vi "CmdReader with Context.vi"() -> ()   [LabVIEW 2020]
doc: "Copyright © 2008 - 2024 VI Technologies B.V. \nALL RIGHTS RESERVED"
uses:
  <vilib>/dex/Stream Element Allocation Mode.ctl
  SuperNS/SuperNS.lvclass
  MsgData/MsgData.lvclass
panel:
  in  "Connection Config":T2={"BufferSize (100)"=100, "Connection Lost Timeout (2000 ms)"=2000, "Element Allocation Mode"=0, "Low latency mode"=enum."None (High througput mode)", "BG ConnCheck/Read period (200 ms)"=200, "OpenProcessWindow"=TRUE} {"Element Allocation Mode" items=["allocate as needed", "pre-allocate"]}
  in  "Remote EP Config":T3
  in  "Local EP Config":cluster{"Context":string, "Name":string}={"Context"="ReadTestEnv", "Name"="ReaderTest"}
  out "Messages":string
  out "error out":errorcluster
  # "Copyright (c) 2024, VI Technologies B.V.\nAll rights reserved.\n\nRedistribution and use in source and binary forms, with or without modification, are permitted provided that \nthe following conditions are met:\n\n * Redistributions of source code must retain the above copyright notice, this list of conditions and the \nfollowing disclaimer.\n * Redistributions in binary form must reproduce the above copyright notice, this list of conditions and the \nfollowing disclaimer in the documentation and/or other materials provided with the distribution.\n * Neither the name of VI Technologies B.V. nor the names of its contributors may be used to endorse or \npromote products derived from this software without specific prior written permission.\n\nTHIS SOFTWARE IS PROVIDED BY THE COPYRIGHT HOLDERS AND CONTRIBUTORS \"AS IS\" AND ANY EXPRESS OR \nIMPLIED WARRANTIES, INCLUDING, BUT NOT LIMITED TO, THE IMPLIED WARRANTIES OF MERCHANTABILITY \nAND FITNESS FOR A PARTICULAR PURPOSE ARE DISCLAIMED. IN NO EVENT SHALL THE COPYRIGHT OWNER OR \nCONTRIBUTORS BE LIABLE FOR ANY DIRECT, INDIRECT, INCIDENTAL, SPECIAL, EXEMPLARY, OR CONSEQUENTIAL \nDAMAGES (INCLUDING, BUT NOT LIMITED TO, PROCUREMENT OF SUBSTITUTE GOODS OR SERVICES; LOSS OF \nUSE, DATA, OR PROFITS; OR BUSINESS INTERRUPTION) HOWEVER CAUSED AND ON ANY THEORY OF LIABILITY, \nWHETHER IN CONTRACT, STRICT LIABILITY, OR TORT (INCLUDING NEGLIGENCE OR OTHERWISE) ARISING IN ANY \nWAY OUT OF THE USE OF THIS SOFTWARE, EVEN IF ADVISED OF THE POSSIBILITY OF SUCH DAMAGE.\n\nFor more information, please visit https://www.vi-tech.nl or contact us at info@vi-tech.nl"
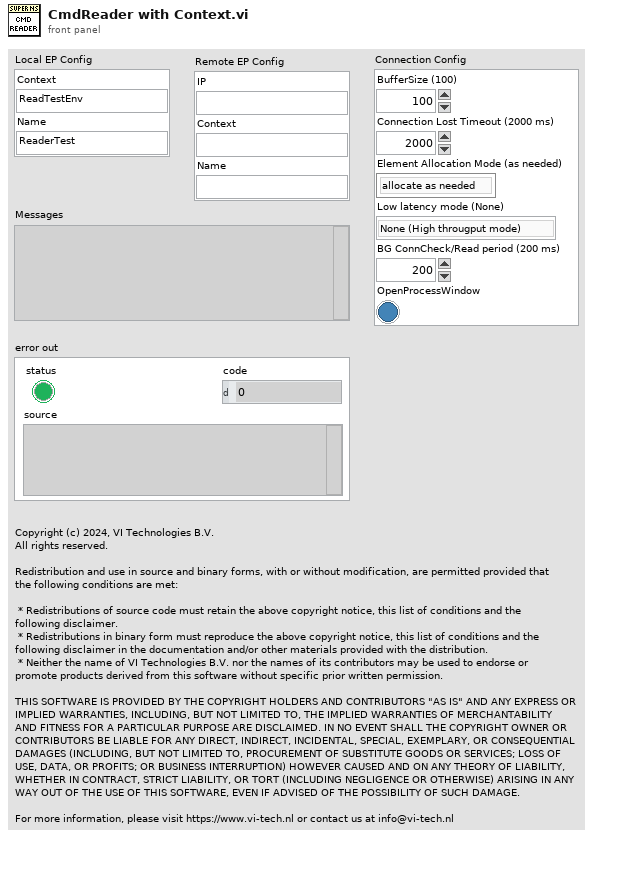
[diagram p1: front panel]
types:
  T1 = typedef "Stream Element Allocation Mode.ctl" = u32
  T2 = cluster{"BufferSize (100)":i32, "Connection Lost Timeout (2000 ms)":i32, "Element Allocation Mode":T1, "Low latency mode":enum16{"None (High througput mode)", "All Elements Read From Stream", "All Elements Available for Reading"}, "BG ConnCheck/Read period (200 ms)":i32, "OpenProcessWindow":bool}
  T3 = cluster{"IP":string, "Context":string, "Name":string}
  T4 = typedef "SuperNS.lvclass/StreamDataType.ctl" = refnum<class>
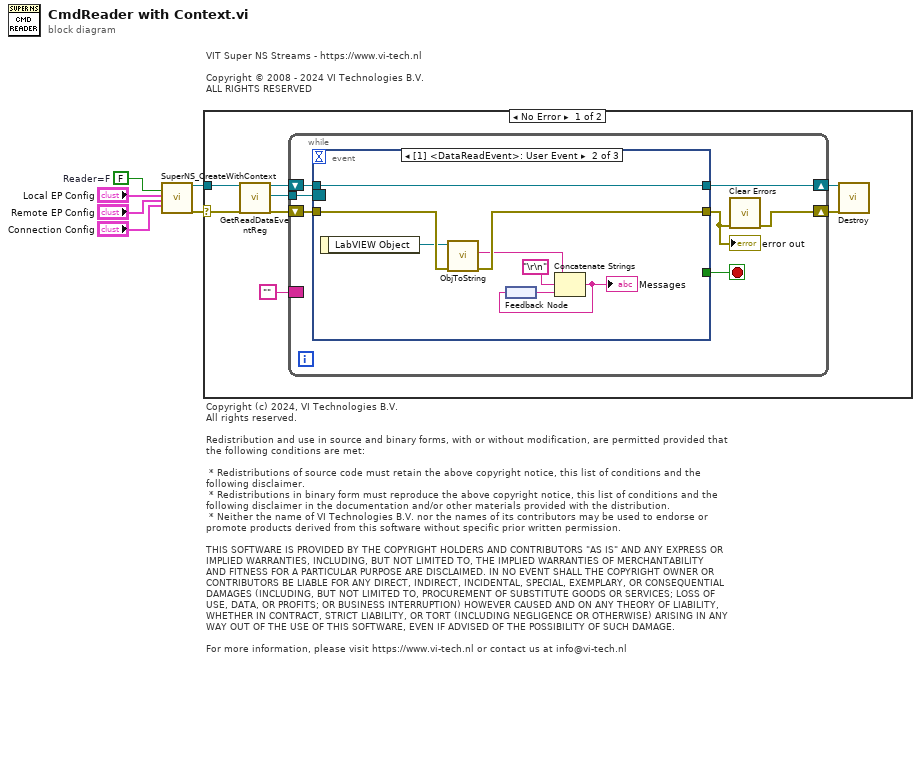
[diagram p0: block diagram]
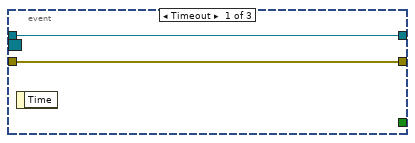
[diagram p2: hidden frame]
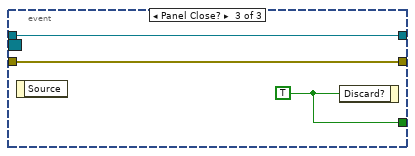
[diagram p3: hidden frame]
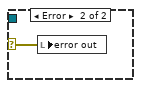
[diagram p4: hidden frame]
diagram:
  w2 = FALSE  # Reader=F
  # "VIT Super NS Streams - https://www.vi-tech.nl\n\nCopyright © 2008 - 2024 VI Technologies B.V. \nALL RIGHTS RESERVED"
  # "Copyright (c) 2024, VI Technologies B.V.\nAll rights reserved.\n\nRedistribution and use in source and binary forms, with or without modification, are permitted provided that \nthe following conditions are met:\n\n * Redistributions of source code must retain the above copyright notice, this list of conditions and the \nfollowing disclaimer.\n * Redistributions in binary form must reproduce the above copyright notice, this list of conditions and the \nfollowing disclaimer in the documentation and/or other materials provided with the distribution.\n * Neither the name of VI Technologies B.V. nor the names of its contributors may be used to endorse or \npromote products derived from this software without specific prior written permission.\n\nTHIS SOFTWARE IS PROVIDED BY THE COPYRIGHT HOLDERS AND CONTRIBUTORS \"AS IS\" AND ANY EXPRESS OR \nIMPLIED WARRANTIES, INCLUDING, BUT NOT LIMITED TO, THE IMPLIED WARRANTIES OF MERCHANTABILITY \nAND FITNESS FOR A PARTICULAR PURPOSE ARE DISCLAIMED. IN NO EVENT SHALL THE COPYRIGHT OWNER OR \nCONTRIBUTORS BE LIABLE FOR ANY DIRECT, INDIRECT, INCIDENTAL, SPECIAL, EXEMPLARY, OR CONSEQUENTIAL \nDAMAGES (INCLUDING, BUT NOT LIMITED TO, PROCUREMENT OF SUBSTITUTE GOODS OR SERVICES; LOSS OF \nUSE, DATA, OR PROFITS; OR BUSINESS INTERRUPTION) HOWEVER CAUSED AND ON ANY THEORY OF LIABILITY, \nWHETHER IN CONTRACT, STRICT LIABILITY, OR TORT (INCLUDING NEGLIGENCE OR OTHERWISE) ARISING IN ANY \nWAY OUT OF THE USE OF THIS SOFTWARE, EVEN IF ADVISED OF THE POSSIBILITY OF SUCH DAMAGE.\n\nFor more information, please visit https://www.vi-tech.nl or contact us at info@vi-tech.nl"
  n1 = call "SuperNS_CreateWithContext.vi"("Writer (F: Reader)"=w2, "Local EP Config"="Local EP Config", "Remote EP Config"="Remote EP Config", "Connection Config"="Connection Config") -> ("reference out"=w5:refnum<class "SuperNS.lvclass">, "error out"=w6:errorcluster)  [unwired: 14 in]
  n2 = case shown="No Error" w6 {
    selector: w6 -> [w13 w35]
    tunnel: w5 -> [w7 _]
    frame No Error {
      n3 = call-dynamic "GetReadDataEventReg.vi"("reference in"=w7, "error in"=w13) -> ("reference out"=w10:refnum<class "SuperNS.lvclass">, "SuperNS ReadData"=w9:refnum<event-registration>, "error out"=w14:errorcluster)  [unwired: 15 in]
      n4 = while {
        shift-right: [w16] -> w11
        shift-left: w10 -> [w17]
        tunnel: w9 -> [w15]
        shift-right: [w20] -> w12
        shift-left: w14 -> [w21]
        border: "" -> [_]
        stop <- w18 stop-if-true
        n5 = event shown="[1] <DataReadEvent>: User Event" {
          selector: w15 -> [_ _ _]
          dyn-events: _ -> [_ _ _]
          timeout: _ -> [_ _ _]
          tunnel: [_ _ w34] -> w18
          tunnel: w17 -> [w23 w29 w33]
          tunnel: [w23 w29 w33] -> w16
          tunnel: w21 -> [w22 w31 w32]
          tunnel: [w22 w30 w32] -> w19
          event Timeout {
            n6 = event-data() -> ()  [unwired: 1 in, 1 out]
          }
          event User Event {
            n7 = event-data() -> ("LabVIEW Object"=w25:T4)  [unwired: 1 in]
            n8 = call "ObjToString.vi"("error in"=w31, "LabVIEW Object"=w25) -> ("error out"=w30:errorcluster, "String"=w24:string)  [unwired: 8 in]
            n9 = feedback #1() -> (w28:string)
            n10 = Concatenate Strings(w24, "\r\n", w28) -> (w26:string)
            "Messages" <- w26
            n11 = feedback-in #1(w26) -> ()
          }
          event Panel Close? {
            w34 = TRUE ("Discard?")
            n12 = event-data() -> ()  [unwired: 1 in, 1 out]
            n13 = event-data("Discard?"=w34) -> ()  [unwired: 1 in, 1 out]
          }
        }
        "error out" <- w19
        n14 = call <vilib>:"Clear Errors.vi"("error in (no error)"=w19) -> ("error out"=w20:errorcluster)  [unwired: 5 in, 1 out]
      }
      n15 = call-dynamic "Destroy.vi"("reference in"=w11, "error in (no error)"=w12) -> ()  [unwired: 16 in, 2 out]
    }
    frame Error {
      n16 = local write "error out"(w35) -> ()
    }
  }
